vi "From Property Object.vi"(8 "error in (no error)":errorcluster, 11 "PropertyObject":refnum<k7>) -> (0 "error out":errorcluster, 3 "VariableContainer":T1)   [LabVIEW 2020]
uses:
  VariableContainer.lvclass
  Typedefs/Session Handle.ctl
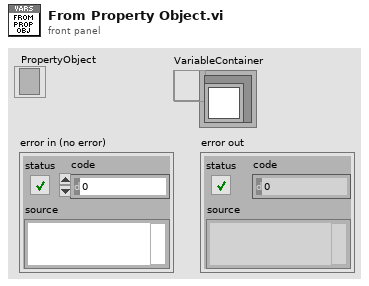
[diagram p1: front panel]
types:
  T1 = typedef "HTS.lvlib/VariableContainer.lvclass/Session Handle.ctl" = refnum<data-value>
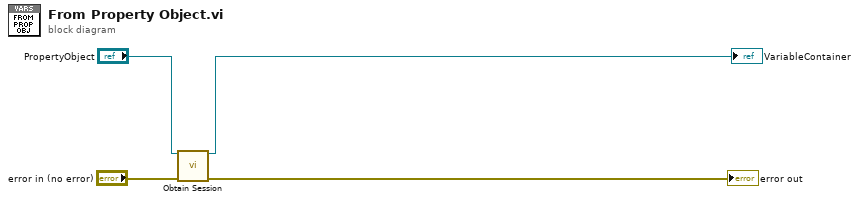
[diagram p0: block diagram]
diagram:
  n1 = call "Obtain Session.vi"("PropertyObject"="PropertyObject", "error in (no error)"="error in (no error)") -> ("Session Handle"=→"VariableContainer":T1, "error out"=→"error out":errorcluster)  [unwired: 12 in]
